vi "Autonomous Independent.vi"() -> ()   [LabVIEW 2017]
doc: "This VI is called when autonomous begins, and will automatically be terminated when autonomous ends. You can carry out timed or sensor driven robot movement independently without needing to return to the caller."
uses:
  <vilib>/Rock Robotics/WPI/Utilities/WPI_GetSetVariantRefNum.vi
  <vilib>/Rock Robotics/Network Tables/NT Read String.vi
  <vilib>/Rock Robotics/Network Tables/NT Write Numeric Array.vi
  Public/Documents/Cross The Road Electronics/Phoenix-LabVIEW/Motor Controller/Get/CTRE_Phoenix_MotorController_GetSelectedSensorData.vi
  <vilib>/Rock Robotics/WPI/RobotDrive/WPI_RobotDriveArcadeDrive_Standard(NoSaturation).vi
panel:
  out "Right Encoder Rotations":dbl format="%.2f"
  out "Right Encoder Inches":dbl format="%.2f"
  out "Right Encoder":i32
  out "Distance (In) Vs. Time":dbl(graph)
  out "Left Encoder Rotations":dbl format="%.2f"
  out "Left Encoder Inchers":dbl format="%.2f"
  out "Left Encoder":i32
  out "Motor Rotations to Travel":dbl
  out "Motor Units to Travel":dbl
  in  "Inchers to Travel":dbl
  # "Be sure to right-click and choose Data Operations>>Make Current Value default if you want to save the array values with the VI"
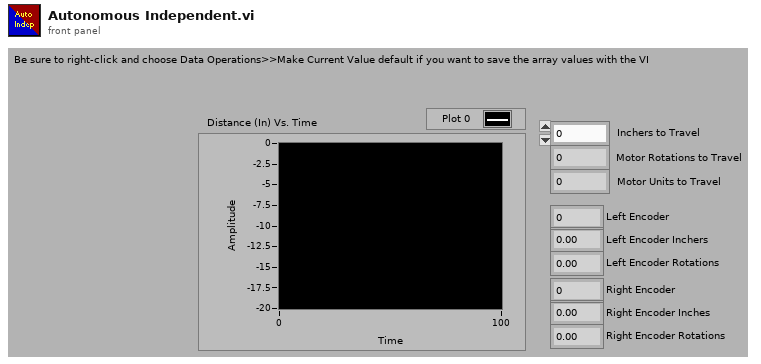
[diagram p1: front panel]
types:
  T1 = typedef "WPI_JoystickDevRef.ctl" = cluster{"Device":T2}
  T2 = typedef "WPI_JoystickDeviceEnum.ctl" = enum16{"USB 0", "USB 1", "USB 2", "USB 3", "USB 4", "USB 5"}
  T3 = typedef "WPI_MotorControlDeviceRef.ctl" = cluster{"DeviceStatus":errorcluster, "Type":T4, "PWM":cluster{"PWM Channel":T5, "DeadBand":T6}, "CAN":cluster{"Device Number":u8, "SetOutput VI Ref":variant, "GetOutput VI Ref":variant, "Enable VI Ref":variant, "Disable VI Ref":variant, "Data":variant}, "Invert":bool, "DIO PWM":cluster{"PWM \"Enable\" Channel":T5, "DIOChannel":T7, "PWM Rate":dbl}}
  T4 = typedef "WPI_MotorControlType.ctl" = enum16{"PWM", "CAN", "DIO PWM"}
  T5 = typedef "FPGA_DIOPWMChannel.ctl" = enum8{"PWM 0", "PWM 1", "PWM 2", "PWM 3", "PWM 4", "PWM 5", "PWM 6", "PWM 7", "PWM 8", "PWM 9", "PWM MXP 0", "PWM MXP 1", "PWM MXP 2", "PWM MXP 3", "PWM MXP 4", "PWM MXP 5", "PWM MXP 6", "PWM MXP 7", "PWM MXP 8", "PWM MXP 9", "Invalid"}
  T6 = typedef "WPI_PWMDeadband.ctl" = cluster{"Name":string, "maxPositivePwm":i32, "minPositivePwm":i32, "centerPwm":i32, "maxNegativePwm":i32, "minNegativePwm":i32, "angularRange":u16}
  T7 = typedef "FPGA_DIOChannel.ctl" = enum8{"DIO 0", "DIO 1", "DIO 2", "DIO 3", "DIO 4", "DIO 5", "DIO 6", "DIO 7", "DIO 8", "DIO 9", "DIO MXP 0", "DIO MXP 1", "DIO MXP 2", "DIO MXP 3", "DIO MXP 4", "DIO MXP 5", "DIO MXP 6", "DIO MXP 7", "DIO MXP 8", "DIO MXP 9", "DIO MXP 10", "DIO MXP 11", "DIO MXP 12", "DIO MXP 13", "DIO MXP 14", "DIO MXP 15", "SPI Port CS1", "SPI Port CS2", "SPI Port CS3", "SPI Port MISO", "SPI Port MOSI", "Invalid"}
  T8 = typedef "WPI_RobotDriveDevRef.ctl" = cluster{"DevStatus":errorcluster, "Motors[]":T3[], "Square Inputs":bool, "Max Output":dbl}
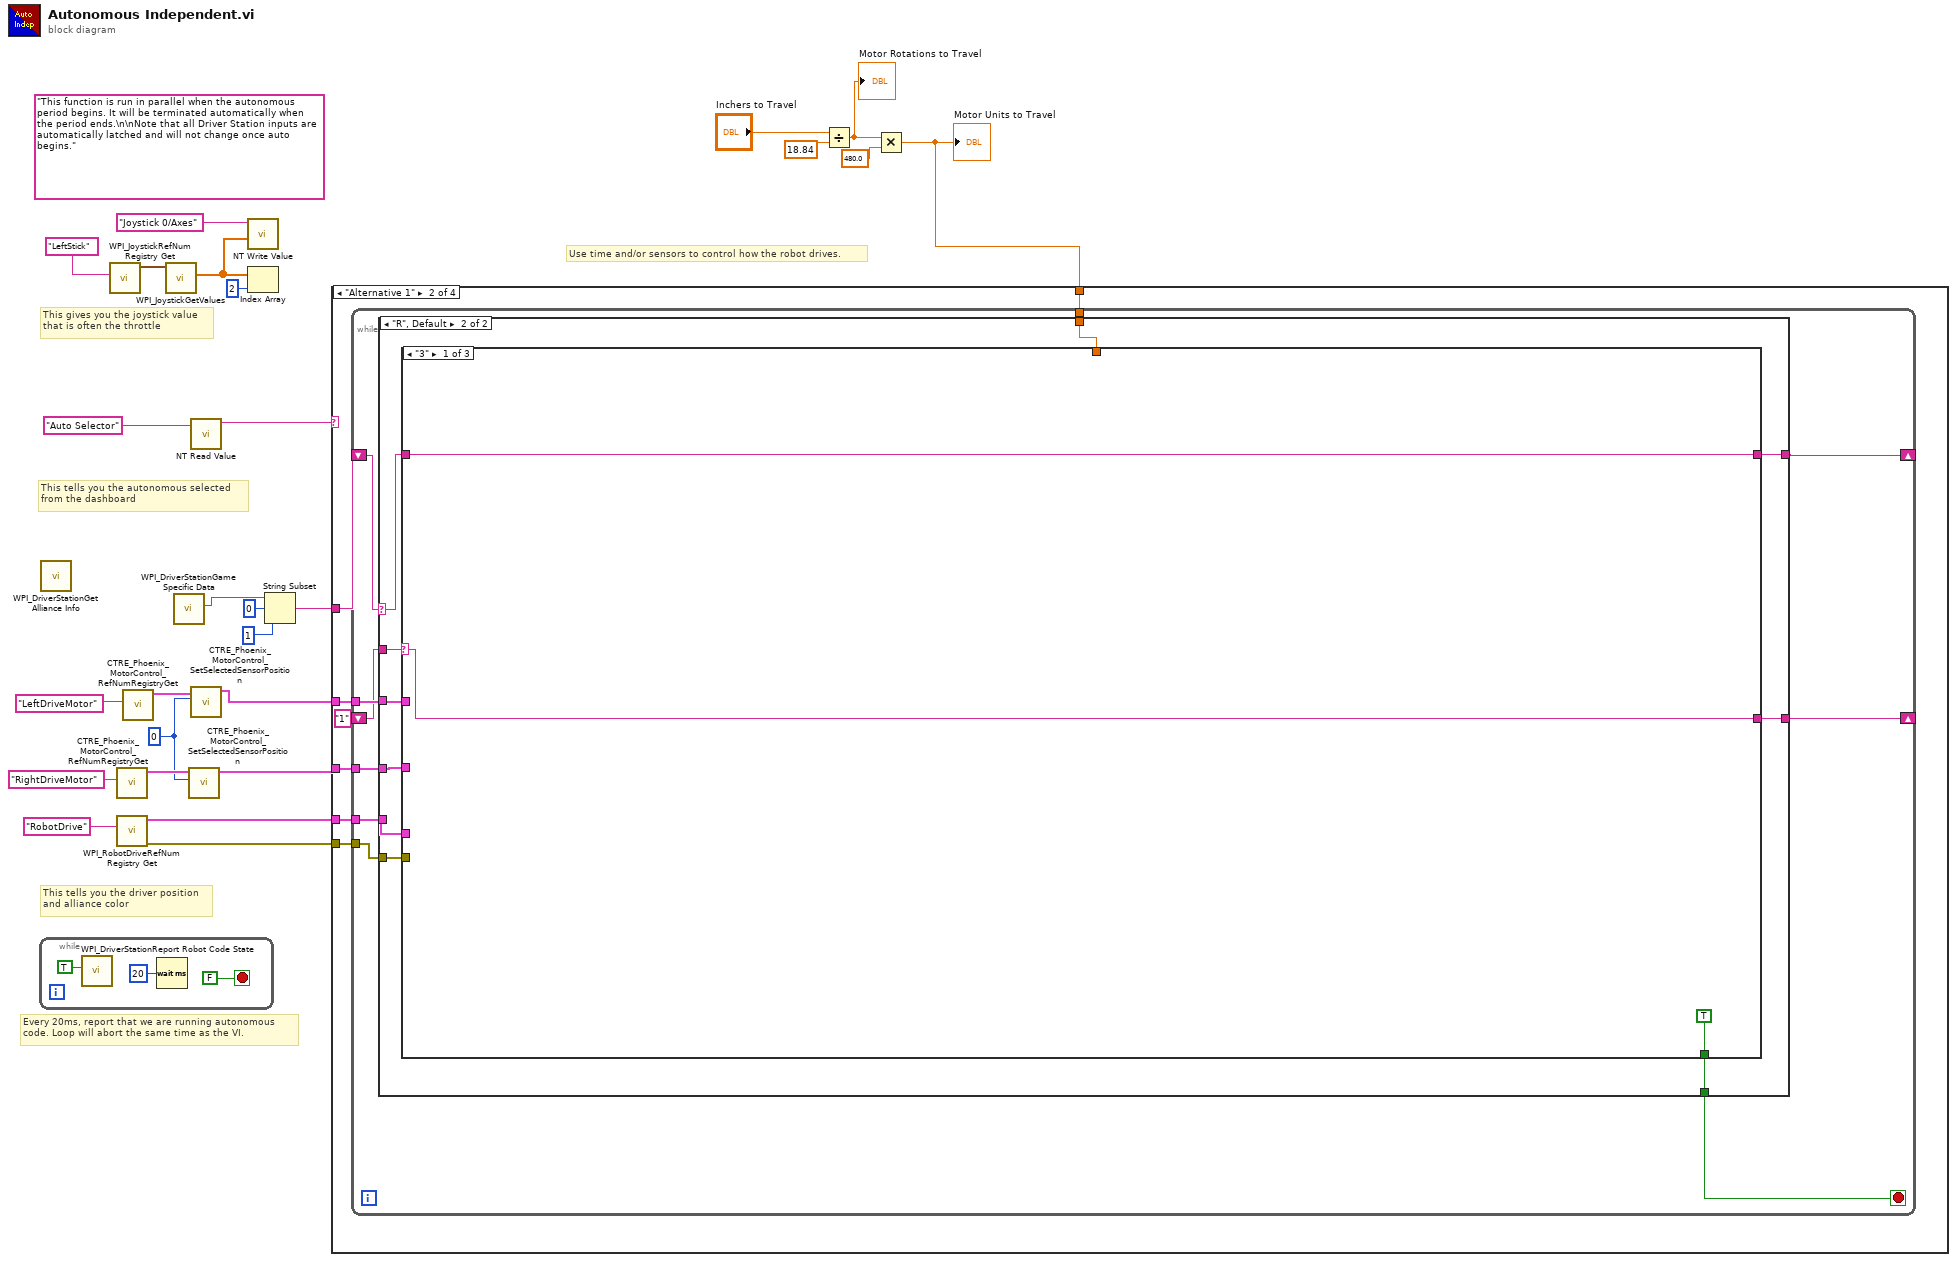
[diagram p0: block diagram]
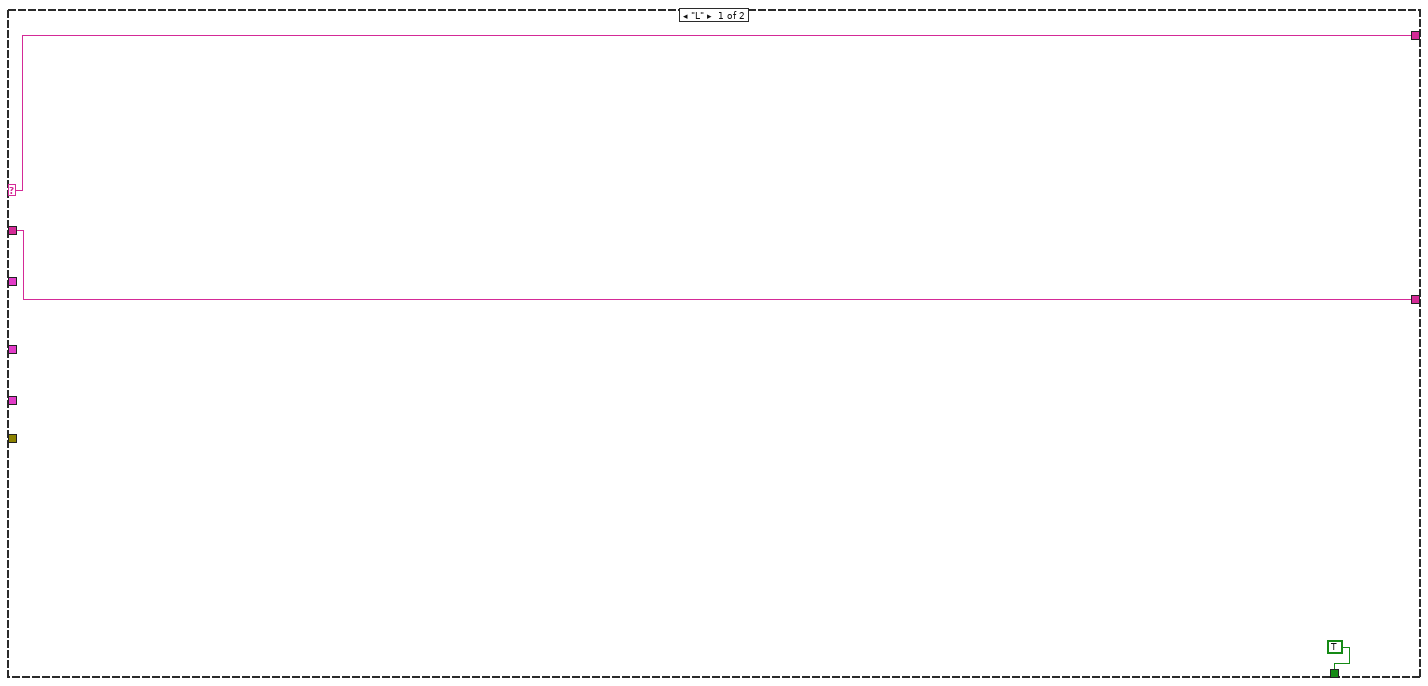
[diagram p3: hidden frame]
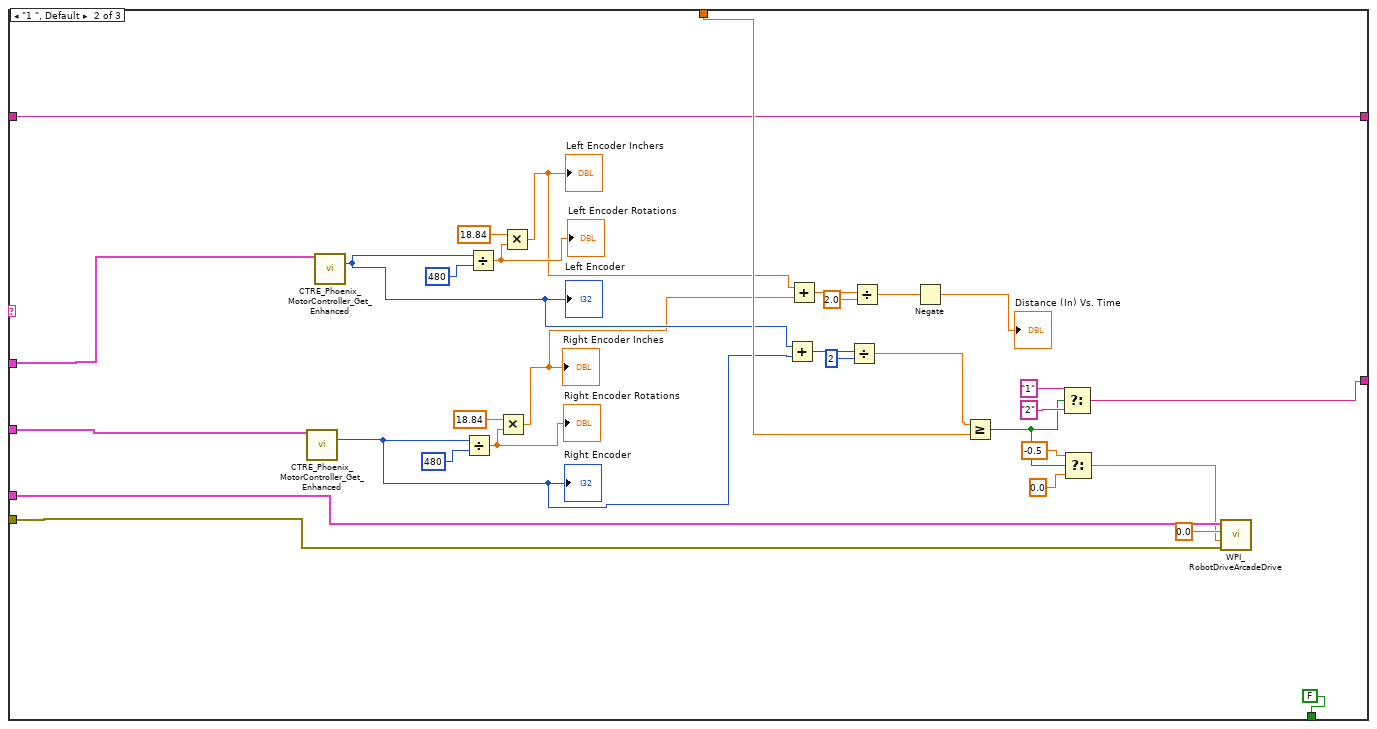
[diagram p4: hidden frame]
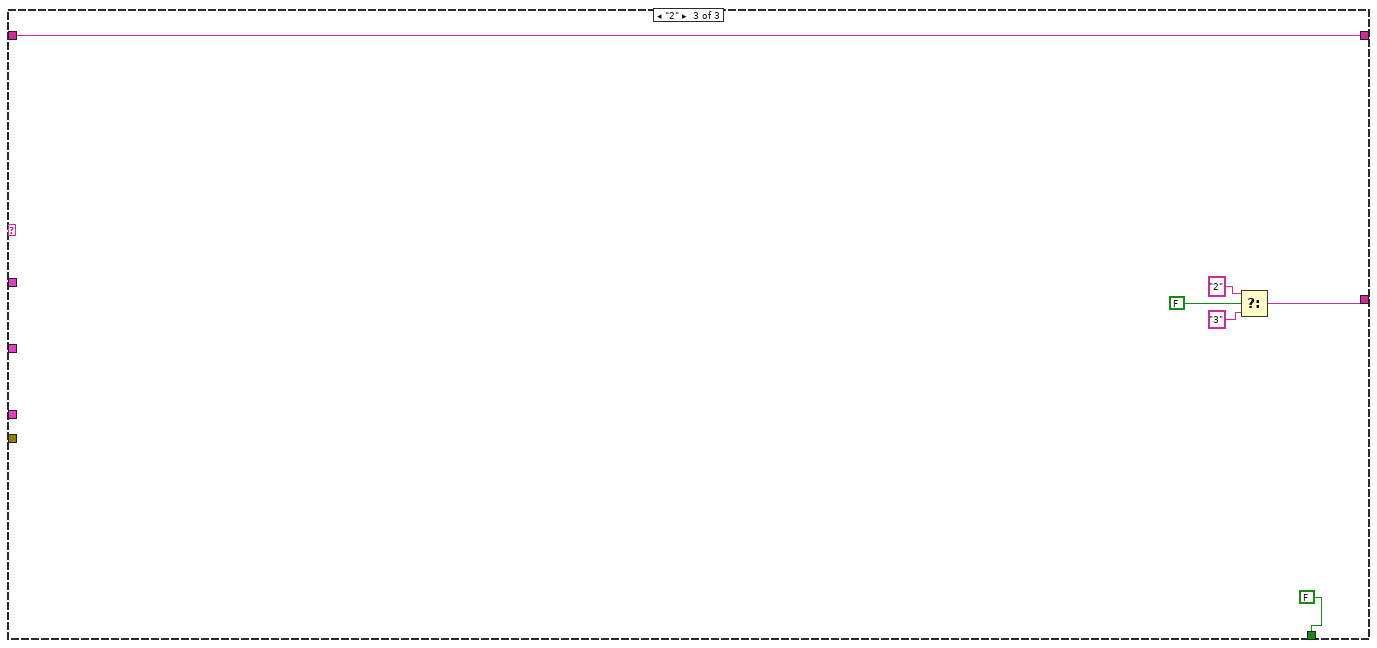
[diagram p5: hidden frame]
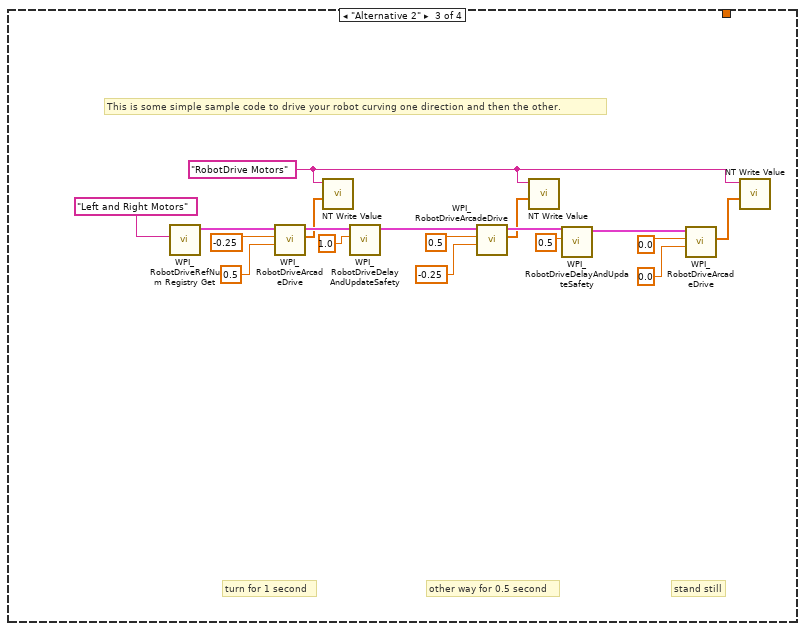
[diagram p6: hidden frame]
diagram:
  w1 = 0 ("New Sensor Position")
  (unwired) "This function is run in parallel when the autonomous period begins. It will be terminated automatically when the period ends.\n\nNote that all Driver Station inputs are automatically latched and will not change once auto begins."
  # "This tells you the autonomous selected\nfrom the dashboard"
  # "Every 20ms, report that we are running autonomous\ncode. Loop will abort the same time as the VI."
  # "This gives you the joystick value\nthat is often the throttle"
  # "Use time and/or sensors to control how the robot drives."
  # "This tells you the driver position\nand alliance color"
  n1 = while {
    stop <- FALSE stop-if-true
    n2 = call <vilib>:"WPI_DriverStationReport Robot Code State.vi"("Autonomous"=TRUE) -> ()  [unwired: 10 in, 1 out]
    n3 = Wait (ms)(milliseconds to wait=u32 20) -> ()  [unwired: 1 out]
  }
  n4 = call <vilib>:"WPI_DriverStationGet Alliance Info.vi"() -> ()  [unwired: 12 out]
  n5 = call <vilib>:"WPI_JoystickRefNum Registry Get.vi"("refnum name"="LeftStick") -> ("JoystickDevRef"=w25:T1)  [unwired: 1 in, 9 out]
  n6 = call "CTRE_Phoenix_MotorControl_RefNumRegistryGet.vi"("refnum name"="RightDriveMotor") -> ("PhoenixMotorControlDevRef"=w3:T3)  [unwired: 9 in, 1 out]
  n7 = call <vilib>:"WPI_RobotDriveRefNum Registry Get.vi"("refnum name"="RobotDrive") -> ("error out"=w6:errorcluster, "RobotDriveDevRef"=w7:T8)  [unwired: 1 in, 8 out]
  n8 = call "CTRE_Phoenix_MotorControl_RefNumRegistryGet.vi"("refnum name"="LeftDriveMotor") -> ("PhoenixMotorControlDevRef"=w5:T3)  [unwired: 9 in, 1 out]
  n9 = call <vilib>:"WPI_JoystickGetValues.vi"("JoystickDevRef"=w25) -> ("Axes"=w21:dbl[])  [unwired: 6 in, 4 out]
  n10 = call <vilib>:"WPI_DriverStationGame Specific Data.vi"() -> ("Game Specific Data"=w19:string)  [unwired: 11 in]
  n11 = call "CTRE_Phoenix_MotorControl_SetSelectedSensorPosition.vi"("New Sensor Position"=w1, "PhoenixMotorControlDevRef"=w3) -> ("PhoenixMotorControlDevRef"=w2:T3)  [unwired: 8 in, 1 out]
  n12 = call-poly <vilib>:"NT Read Value.vi"("Name"="Auto Selector") -> ("String"=w22:string)  [unwired: 9 in, 1 out]
  n13 = call "CTRE_Phoenix_MotorControl_SetSelectedSensorPosition.vi"("New Sensor Position"=w1, "PhoenixMotorControlDevRef"=w5) -> ("PhoenixMotorControlDevRef"=w4:T3)  [unwired: 8 in, 1 out]
  n14 = call-poly <vilib>:"NT Write Value.vi"("Numeric Array"=w21, "Name"="Joystick 0/Axes") -> ()  [unwired: 9 in, 1 out]
  n15 = Index Array(array=w21, index=2) -> ()  [unwired: 1 out]
  n16 = String Subset(string=w19, offset (0)=0, length (rest)=1 ("length (rest)")) -> (substring=w16:string)
  n17 = Divide(x="Inchers to Travel", y=18.84) -> (x/y=w12:dbl)
  "Motor Rotations to Travel" <- w12
  n18 = Multiply(x=w12, y=480.0) -> (x*y=w11:dbl)
  "Motor Units to Travel" <- w11
  n19 = case shown="\"Alternative 1\"" w22 {
    tunnel: w16 -> [_ w31 _ _]
    tunnel: w11 -> [_ w36 _ _]
    tunnel: w2 -> [_ w32 _ _]
    tunnel: w4 -> [_ w35 _ _]
    tunnel: w7 -> [_ w34 _ _]
    tunnel: w6 -> [_ w33 _ _]
    frame Default {
      # "You can put your main auto here, or you can right-click on the case and make any\nother frame be the default case."
      # "This is the frame that will execute if no selection is made, or if it is not recognized"
    }
    frame "Alternative 1" {
      n20 = while {
        tunnel: w36 -> [w46]
        tunnel: w35 -> [w45]
        tunnel: w34 -> [w44]
        tunnel: w33 -> [w43]
        tunnel: w32 -> [w42]
        shift-right: [w41] -> _
        shift-left: w31 -> [w40]
        shift-right: [w39] -> _
        shift-left: "1" -> [w38]
        stop <- w37 stop-if-true
        n21 = case shown="\"R\", Default" w40 {
          selector: w40 -> [w49 w53]
          tunnel: w45 -> [_ w57]
          tunnel: w46 -> [_ w55]
          tunnel: w42 -> [_ w56]
          tunnel: w44 -> [_ w59]
          tunnel: w43 -> [_ w58]
          tunnel: [w49 w54] -> w41
          tunnel: [w48 w52] -> w39
          tunnel: w38 -> [w48 w51]
          tunnel: [TRUE w50] -> w37
          frame "L" {
          }
          frame "R", Default {
            n22 = case shown="\"3\"" w51 {
              selector: w51 -> [w61 _ _]
              tunnel: w59 -> [_ w94 _]
              tunnel: w58 -> [_ w93 _]
              tunnel: w57 -> [_ w92 _]
              tunnel: w56 -> [_ w91 _]
              tunnel: w55 -> [_ w90 _]
              tunnel: w53 -> [w62 w89 w100]
              tunnel: [w62 w89 w100] -> w54
              tunnel: [w61 w67 w96] -> w52
              tunnel: [TRUE FALSE FALSE] -> w50
              frame "3" {
              }
              frame "1 ", Default {
                n23 = call-poly "CTRE_Phoenix_MotorController_Get_Enhanced.vi"("PhoenixMotorControlDevRef"=w91) -> ("Position (Raw Sensor Units)"=w79:i32)  [unwired: 11 in, 3 out]
                "Right Encoder" <- w79
                n24 = call-poly "CTRE_Phoenix_MotorController_Get_Enhanced.vi"("PhoenixMotorControlDevRef"=w92) -> ("Position (Raw Sensor Units)"=w80:i32)  [unwired: 11 in, 3 out]
                "Left Encoder" <- w80
                n25 = Divide(x=w79, y=480) -> (x/y=w81:dbl)
                "Right Encoder Rotations" <- w81
                n26 = Divide(x=w80, y=480) -> (x/y=w84:dbl)
                "Left Encoder Rotations" <- w84
                n27 = Multiply(x=18.84, y=w81) -> (x*y=w75:dbl)
                "Right Encoder Inches" <- w75
                n28 = Multiply(x=18.84, y=w84) -> (x*y=w74:dbl)
                "Left Encoder Inchers" <- w74
                n29 = Add(x=w80, y=w79) -> (x+y=w78:i32)
                n30 = Add(x=w74, y=w75) -> (x+y=w73:dbl)
                n31 = Divide(x=w78, y=2) -> (x/y=w76:dbl)
                n32 = Divide(x=w73, y=2.0) -> (x/y=w71:dbl)
                n33 = Negate(x=w71) -> (-x=→"Distance (In) Vs. Time":dbl)
                n34 = Greater Or Equal?(x=w76, y=w90) -> (x >= y?=w66:bool)
                n35 = Select(t="1", s=w66, f="2") -> (s? t:f=w67:string)
                n36 = Select(t=-0.5, s=w66, f=0.0) -> (s? t:f=w63:dbl)
                n37 = call-poly <vilib>:"WPI_RobotDriveArcadeDrive.vi"("error in (no error)"=w93, "Y axis value"=w63, "X axis value"=0.0, "RobotDriveDevRef"=w94) -> ()  [unwired: 5 in, 3 out]
              }
              frame "2" {
                n38 = Select(t="2", s=FALSE, f="3") -> (s? t:f=w96:string)
              }
            }
          }
        }
      }
    }
    frame "Alternative 2" {
      w102 = "RobotDrive Motors" ("Name")
      # "This is some simple sample code to drive your robot curving one direction and then the other."
      # "stand still"
      # "other way for 0.5 second"
      # "turn for 1 second"
      n39 = call <vilib>:"WPI_RobotDriveRefNum Registry Get.vi"("refnum name"="Left and Right Motors") -> ("RobotDriveDevRef"=w118:T8)  [unwired: 1 in, 9 out]
      n40 = call-poly <vilib>:"WPI_RobotDriveArcadeDrive.vi"("Y axis value"=0.5 ("X axis value"), "X axis value"=-0.25, "RobotDriveDevRef"=w118) -> ("Motor Values"=w101:dbl[], "RobotDriveDevRef"=w111:T8)  [unwired: 1 in, 6 out]
      n41 = call-poly <vilib>:"NT Write Value.vi"("Numeric Array"=w101, "Name"=w102) -> ()  [unwired: 9 in, 1 out]
      n42 = call <vilib>:"WPI_RobotDriveDelayAndUpdateSafety.vi"("Delay (s)"=1.0, "RobotDriveDevRef"=w111) -> ("RobotDriveDevRef 2"=w112:T8)  [unwired: 8 in, 1 out]
      n43 = call-poly <vilib>:"WPI_RobotDriveArcadeDrive.vi"("Y axis value"=-0.25 ("X axis value"), "X axis value"=0.5, "RobotDriveDevRef"=w112) -> ("Motor Values"=w103:dbl[], "RobotDriveDevRef"=w113:T8)  [unwired: 1 in, 6 out]
      n44 = call-poly <vilib>:"NT Write Value.vi"("Numeric Array"=w103, "Name"=w102) -> ()  [unwired: 9 in, 1 out]
      n45 = call <vilib>:"WPI_RobotDriveDelayAndUpdateSafety.vi"("Delay (s)"=0.5, "RobotDriveDevRef"=w113) -> ("RobotDriveDevRef 2"=w114:T8)  [unwired: 8 in, 1 out]
      n46 = call-poly <vilib>:"WPI_RobotDriveArcadeDrive.vi"("Y axis value"=0.0 ("X axis value"), "X axis value"=0.0, "RobotDriveDevRef"=w114) -> ("Motor Values"=w104:dbl[])  [unwired: 1 in, 7 out]
      n47 = call-poly <vilib>:"NT Write Value.vi"("Numeric Array"=w104, "Name"=w102) -> ()  [unwired: 9 in, 1 out]
    }
    frame "Your Turn" {
    }
  }
